vi "Raw Script.vi"() -> ()   [LabVIEW 2026]
uses:
  <vilib>/Utility/sysdir.llb/System Directory Type.ctl
  <extravilib>/ChannelInstances/Tag-bool/Read With Abort.vi
  <extravilib>/ChannelInstances/Tag-bool/Write With Abort.vi
  <extravilib>/ChannelInstances/Tag-bool/Instantiate.vi
  <extravilib>/ChannelInstances/Tag-bool/EndpointRead.vi
  <extravilib>/ChannelInstances/Tag-bool/Endpoint.vi
  <extravilib>/ChannelInstances/Tag-bool.lvlib
panel:
  out "Banner Text":bool
  out "Command Output":string="Loading..."
  # "After synchronization is complete, be sure to launch the VIDEO GUIDE on the desktop to begin your evaluation.\n\nMultiple resources for your evaluation are laid out in detail.\n\n'Dimension of Evaluation' accompanies the video content\n\nNOTE: Only files saved in 'HOME FOLDER' will be retained in-case-of disconnection"
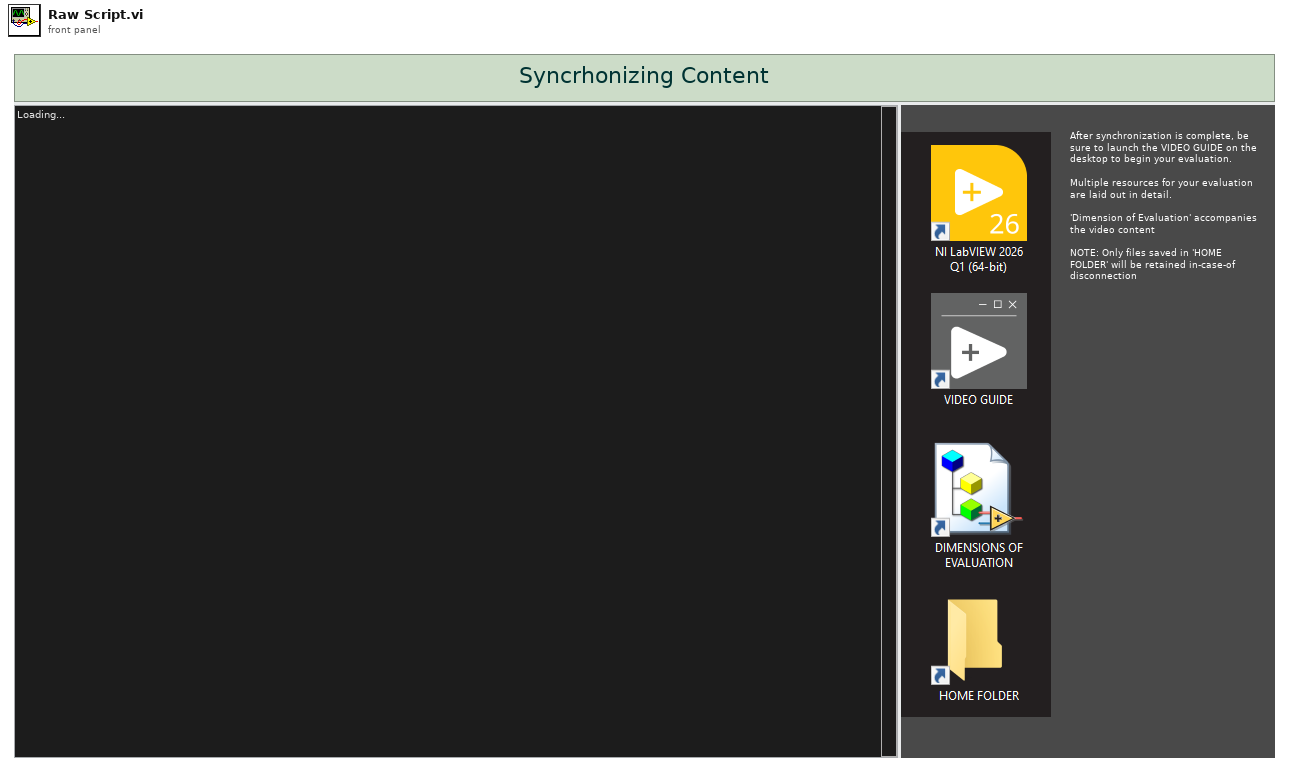
[diagram p1: front panel]
types:
  T1 = typedef "System Directory Type.ctl" = i32
  T2 = typedef "Tag-bool.lvlib/))Channel.ctl" = refnum<queue>
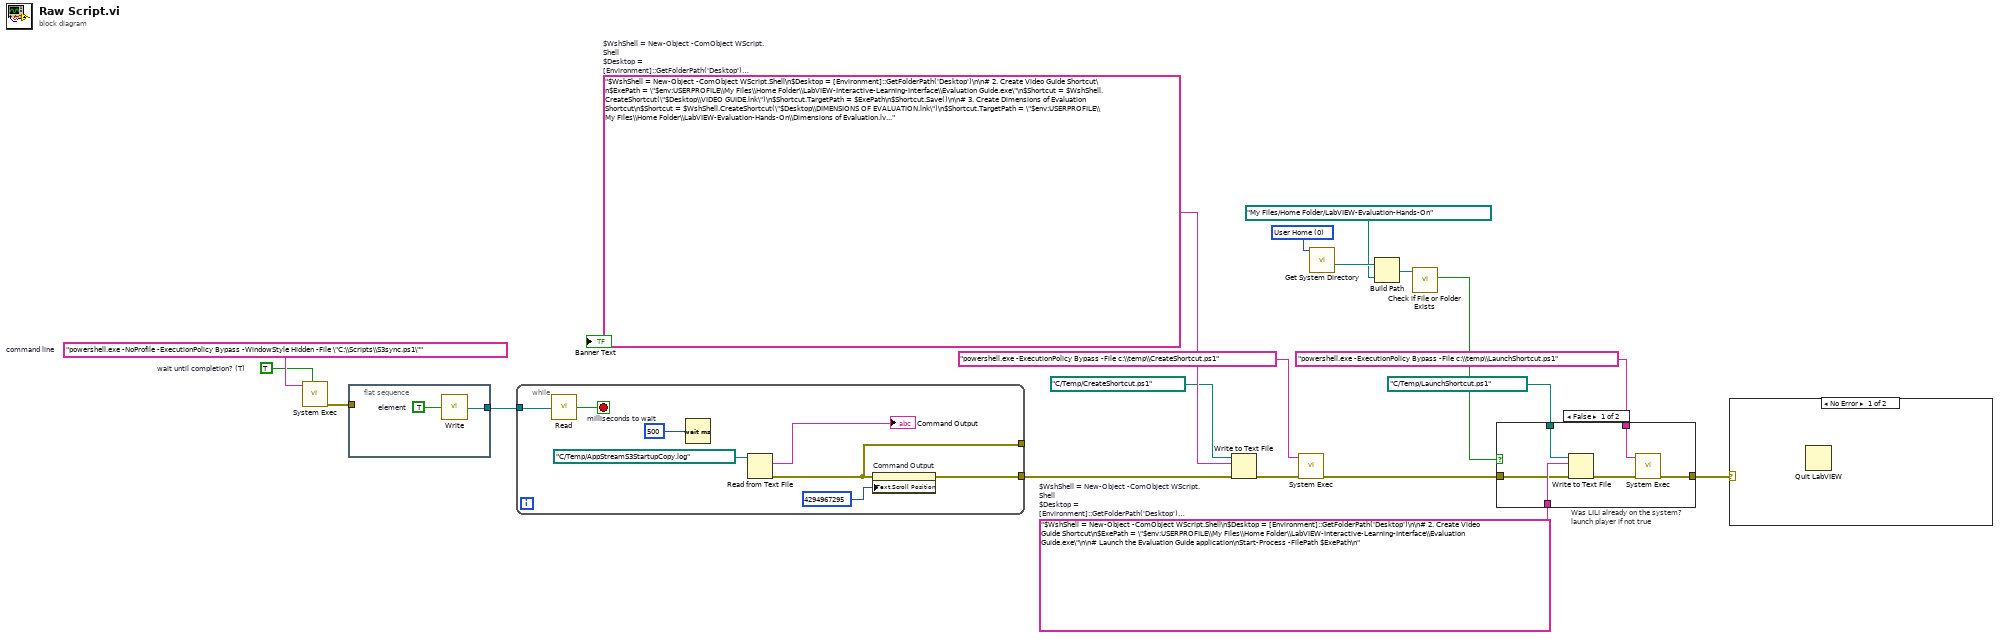
[diagram p0: block diagram]
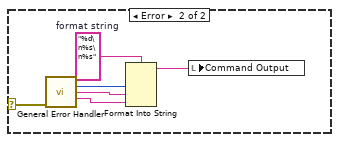
[diagram p2: hidden frame]
diagram:
  w2 = T1 0 items=["User Home"=0, "User Desktop"=1, "User Documents"=2, "User Application Data"=3, "User Preferences"=4, "User Temporary"=5, "Public Documents"=6, "Public Application Data"=7, "Public Preferences"=8, "Public Cache"=13, "System Core Libraries"=9, "System Installed Libraries"=10, "Application Files"=11, "Boot Volume Root"=12] ("system directory type")
  w8 = "$WshShell = New-Object -ComObject WScript.Shell\n$Desktop = [Environment]::GetFolderPath('Desktop')\n\n# 2. Create Video Guide Shortcut\n$ExePath = \"$env:USERPROFILE\\My Files\\Home Folder\\LabVIEW-Interactive-Learning-Interface\\Evaluation Guide.exe\"\n\n# Launch the Evaluation Guide application\nStart-Process -FilePath $ExePath\n"  # $WshShell = New-Object -ComObject WScript.Shell $Desktop = [Environment]::GetFolderPath('Desktop')  # 2. Create Video Guide Shortcut $ExePath = "$env:USERPROFILE\My Files\Home Folder\LabVIEW-Interactive-Learning-Interface\Evaluation Guide.exe"  # Launch the Evaluation Guide application Start-Process -FilePath $ExePath
  w15 = "$WshShell = New-Object -ComObject WScript.Shell\n$Desktop = [Environment]::GetFolderPath('Desktop')\n\n# 2. Create Video Guide Shortcut\n$ExePath = \"$env:USERPROFILE\\My Files\\Home Folder\\LabVIEW-Interactive-Learning-Interface\\Evaluation Guide.exe\"\n$Shortcut = $WshShell.CreateShortcut(\"$Desktop\\VIDEO GUIDE.lnk\")\n$Shortcut.TargetPath = $ExePath\n$Shortcut.Save()\n\n# 3. Create Dimensions of Evaluation Shortcut\n$Shortcut = $WshShell.CreateShortcut(\"$Desktop\\DIMENSIONS OF EVALUATION.lnk\")\n$Shortcut.TargetPath = \"$env:USERPROFILE\\My Files\\Home Folder\\LabVIEW-Evaluation-Hands-On\\Dimensions of Evaluation.lvproj\"\n$Shortcut.Save()\n\n# 1. Create Home Folder Shortcut\n$Shortcut = $WshShell.CreateShortcut(\"$Desktop\\HOME FOLDER.lnk\")\n$Shortcut.TargetPath = \"$env:USERPROFILE\\My Files\\Home Folder\\\"\n$Shortcut.Save()\n\n\n\n"  # $WshShell = New-Object -ComObject WScript.Shell $Desktop = [Environment]::GetFolderPath('Desktop')  # 2. Create Video Guide Shortcut $ExePath = "$env:USERPROFILE\My Files\Home Folder\LabVIEW-Interactive-Learning-Interface\Evaluation Guide.exe" $Shortcut = $WshShell.CreateShortcut("$Desktop\VIDEO GUIDE.lnk") $Shortcut.TargetPath = $ExePath $Shortcut.Save()  # 3. Create Dimensions of Evaluation Shortcut $Shortcut = $WshShell.CreateShortcut("$Desktop\DIMENSIONS OF EVALUATION.lnk") $Shortcut.TargetPath = "$env:USERPROFILE\My Files\Home Folder\LabVIEW-Evaluation-Hands-On\Dimensions of Evaluation.lvproj" $Shortcut.Save()  # 1. Create Home Folder Shortcut $Shortcut = $WshShell.CreateShortcut("$Desktop\HOME FOLDER.lnk") $Shortcut.TargetPath = "$env:USERPROFILE\My Files\Home Folder\" $Shortcut.Save()
  w18 = TRUE  # wait until completion? (T)
  w19 = "powershell.exe -NoProfile -ExecutionPolicy Bypass -WindowStyle Hidden -File \"C:\\Scripts\\S3sync.ps1\""  # command line
  n1 = call <vilib>:"System Exec.vi"("wait until completion? (T)"=w18, "command line"=w19) -> ("error out"=w16:errorcluster)  [unwired: 6 in, 3 out]
  n2 = flat-sequence {
    tunnel: [w20] -> w17
    tunnel: w16 -> [_]
    frame #0 {
      w21 = TRUE  # element
      n3 = call <extravilib>:"Write.vi"("element"=w21) -> ("channel"=w20:T2)  [unwired: 1 out]
    }
  }
  n4 = while {
    tunnel: w17 -> [w27]
    tunnel: [w24] -> _
    tunnel: [w22] -> w11
    stop <- w26 stop-if-true
    w23 = u32 500  # milliseconds to wait
    n5 = call <extravilib>:"Read.vi"("channel"=w27) -> ("element"=w26:bool)  [unwired: 1 in, 1 out]
    n6 = Wait (ms)(milliseconds to wait=w23) -> ()  [unwired: 1 out]
    n7 = Read from Text File(file (use dialog)=path "C:/Temp/AppStreamS3StartupCopy.log") -> (text=→"Command Output":string, error out=w24:errorcluster)  [unwired: 3 in, 2 out]
    n8 = property on="Command Output" class="Str"(error in=w24, "Text.Scroll Position"=u32 4294967295) -> (error out=w22:errorcluster)  [unwired: 1 in, 1 out]
  }
  n9 = Write to Text File(file (use dialog)=path "C:/Temp/CreateShortcut.ps1", text=w15, error in=w11) -> (error out=w12:errorcluster)  [unwired: 1 in, 2 out]
  n10 = call <vilib>:"System Exec.vi"("error in (no error)"=w12, "command line"="powershell.exe -ExecutionPolicy Bypass -File c:\\temp\\CreateShortcut.ps1") -> ("error out"=w7:errorcluster)  [unwired: 6 in, 3 out]
  n11 = call <vilib>:"Get System Directory.vi"("system directory type"=w2) -> ("system directory"=w5:path)  [unwired: 10 in]
  n12 = Build Path(base path=w5, name or relative path=path "My Files/Home Folder/LabVIEW-Evaluation-Hands-On") -> (appended path=w3:path)
  n13 = call <vilib>:"Check if File or Folder Exists.vi"("path"=w3) -> ("file or folder exists?"=w6:bool)  [unwired: 8 in, 2 out]
  n14 = case "Was LILI already on the system? \nlaunch player if not true" shown="False" w6 {
    tunnel: "powershell.exe -ExecutionPolicy Bypass -File c:\\temp\\LaunchShortcut.ps1" -> [w34 _]
    tunnel: path "C:/Temp/LaunchShortcut.ps1" -> [w33 _]
    tunnel: w8 -> [w32 _]
    tunnel: w7 -> [w31 w36]
    tunnel: [w30 w36] -> w1
    frame False {
      n15 = Write to Text File(file (use dialog)=w33, text=w32, error in=w31) -> (error out=w35:errorcluster)  [unwired: 1 in, 2 out]
      n16 = call <vilib>:"System Exec.vi"("error in (no error)"=w35, "command line"=w34) -> ("error out"=w30:errorcluster)  [unwired: 6 in, 3 out]
    }
    frame True {
    }
  }
  n17 = case shown="No Error" w1 {
    selector: w1 -> [_ w42]
    frame No Error {
      n18 = Quit LabVIEW() -> ()  [unwired: 1 in]
    }
    frame Error {
      w37 = "%d\n%s\n%s"  # format string
      n19 = call <vilib>:"General Error Handler.vi"("error in (no error)"=w42) -> ("code out"=w41:i32, "source out"=w40:string, "message"=w39:string)  [unwired: 10 in, 2 out]
      n20 = Format Into String(format string=w37, w41, w40, w39) -> (resulting string=w38:string)  [unwired: 2 in, 1 out]
      n21 = local write "Command Output"(w38) -> ()
    }
  }
